vi "pih.hReadChannels-UandP-2018.vi"(0 "FPGA VI Reference In":refnum<k20>, 2 "SampleTime":sgl=0.0004, 3 "final channel selection":i64[][](array[numeric]), 4 "kbolott_and_volume":sgl[][](array[numeric]), 5 "Nsamples":u32, 7 "error in":errorcluster, 8 "Tau/dt":sgl[](array[numeric]), 9 "Scale(mV)":sgl[](array[numeric]), 11 "av power array":refnum<vi>, 15 "RawScal":sgl[](array[numeric]), 16 "SumScal":sgl[](array[numeric]), 17 "current P_rad sample":refnum<vi>) -> (1 "Fehler":bool, 20 "FPGA VI Reference Out":refnum<k20>, 21 "PowerArray":sgl[][](array[numeric]), 25 "RawArray":sgl[][](array[numeric]), 27 "error out":errorcluster)   [LabVIEW 2014]
doc: "startet das einlesen und führt dies bis n Samples aus\nHier mit FIFO und IRQ."
uses:
  <vilib>/Utility/error.llb/Error Cluster From Error Code.vi
  <vilib>/rvi/errors/niLvFpgaAdjustHostInterfaceError.vi
  <vilib>/RVI Host/nirviSupport.llb/nirviErrorClusterFromErrorCode.vi
  <vilib>/rvi/interface/nirviReadWriteControl/nirviReadWriteControl.xnode
  FPGA Bitfiles/W7XBolo2017_FPGATarget_fmain2014_9xlV3GyHFfo.lvbitx
  f_main_2014.vi
  <vilib>/rvi/interface/nirviMethod/nirviMethod.xnode
  NiFpgaLv.dll
  <vilib>/rvi/interface/nirviMethod/StockFPGA_InlinedMethodWaitForMultipleIRQ.vi
  <vilib>/FPGAPlugInAG/PCI-7813R/niLvFpga_WaitOnIrq_PCI-7813R.vi
  <vilib>/FPGAPlugInAG/PCI-7813R/niLvFpga_AcknowledgeIrq_PCI-7813R.vi
  <vilib>/FPGAPlugInAG/PCI-7813R/niLvFpga_ReadFifo_PCI-7813R.vi
  <vilib>/rvi/errors/niLvFpgaMergeErrorWithErrorCode.vi
panel:
  out "Array":sgl[](array[numeric])
  out "last sample":sgl[](array[numeric])
  out "x*2^n":dbl[](array[numeric])
  out "av array":dbl[](array[numeric])
  out "V_Cam":dbl format="%#_13g"
  out "new level of override":i32
  out "rt prad average array":dbl[][](array[numeric])
  out "rawarray":sgl[][](array[numeric])
  out "powerarray":sgl[][](array[numeric])
  out "current sample array":sgl[](array[numeric])
  in  "wait ms":i32
  out "column":i32
  out "channel index":i32
  out "sample":i32
  out "current P_rad [MW]":dbl
  out "elec. channel selected":i64
  out "sate":string
  out "element of channel\nand sample":sgl
  out "channel number":i64
  out "Elements Remaining":u32
  out "STOP?":bool
  out "Timed Out":bool
  # "Sampling"
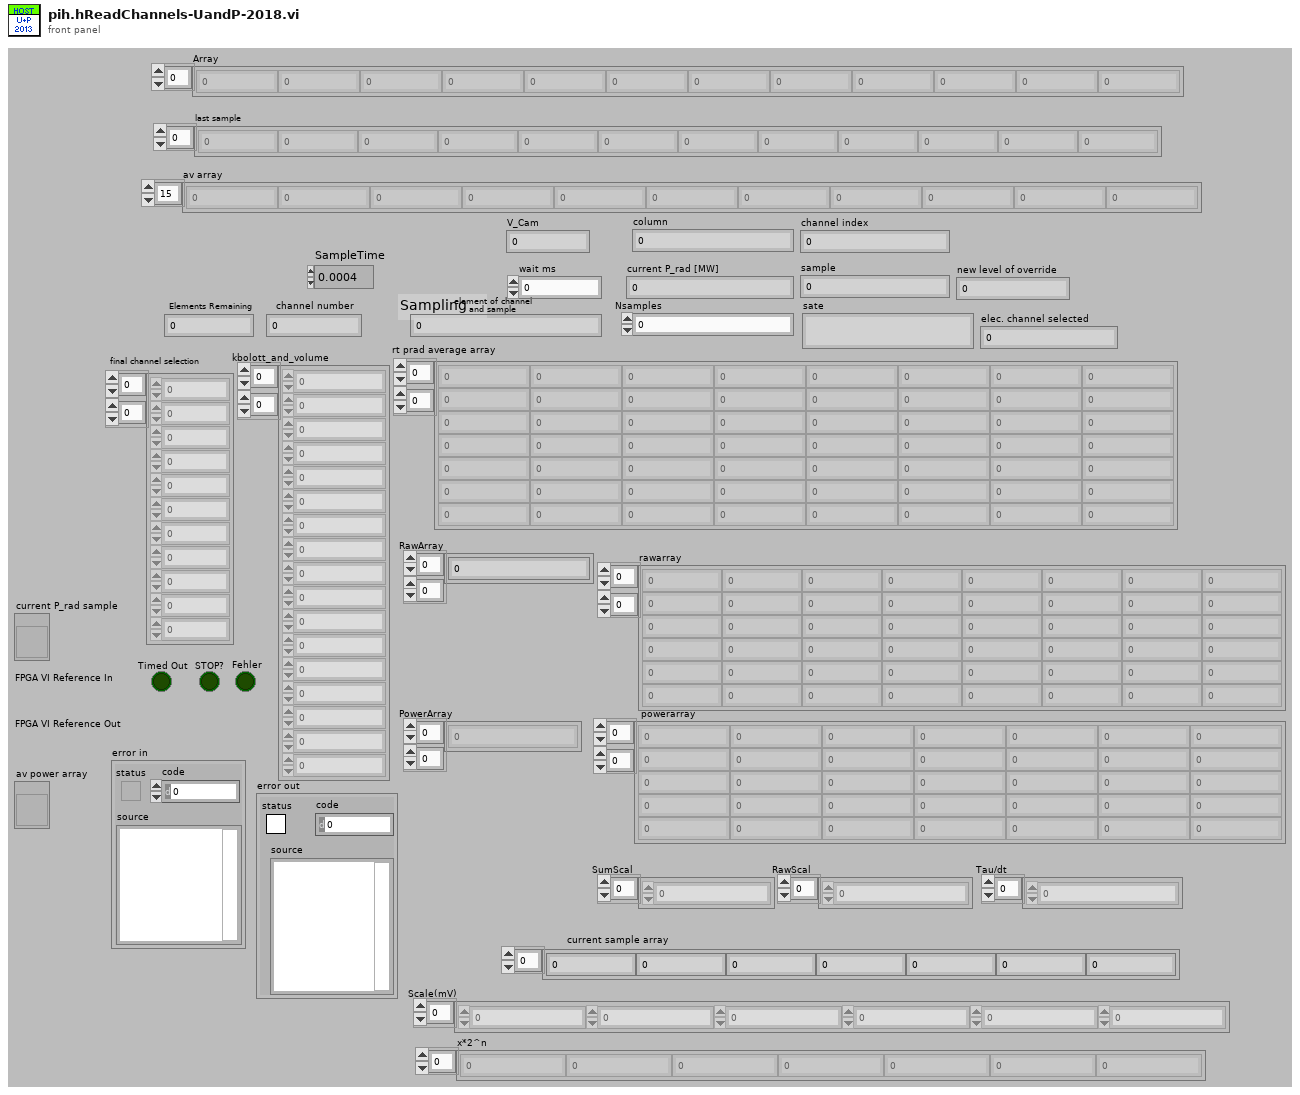
[diagram p1: front panel]
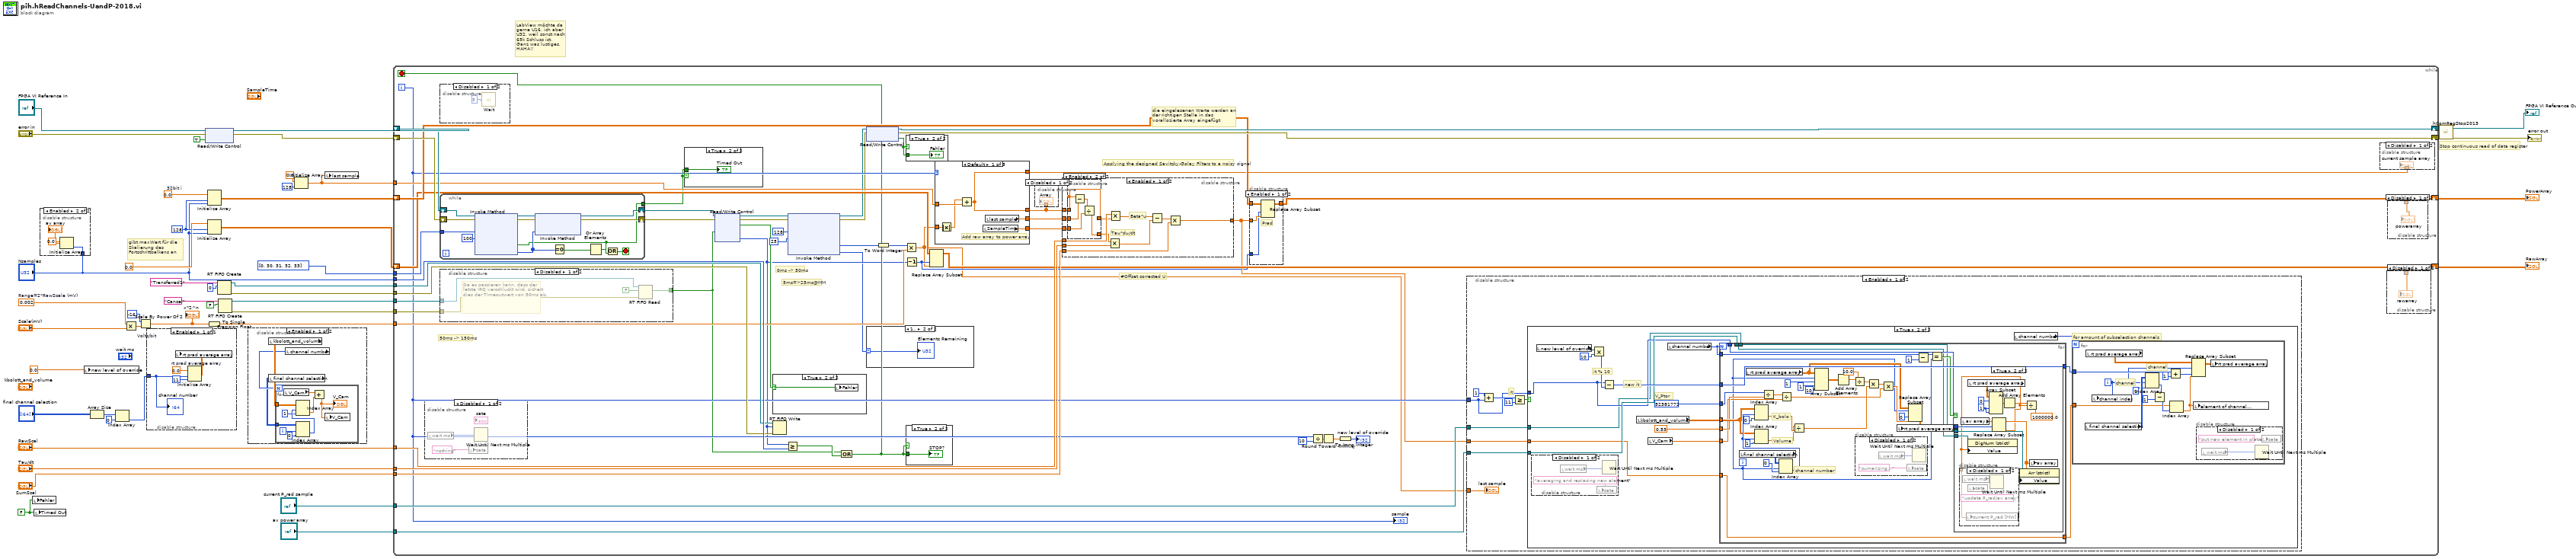
[diagram p0: block diagram]
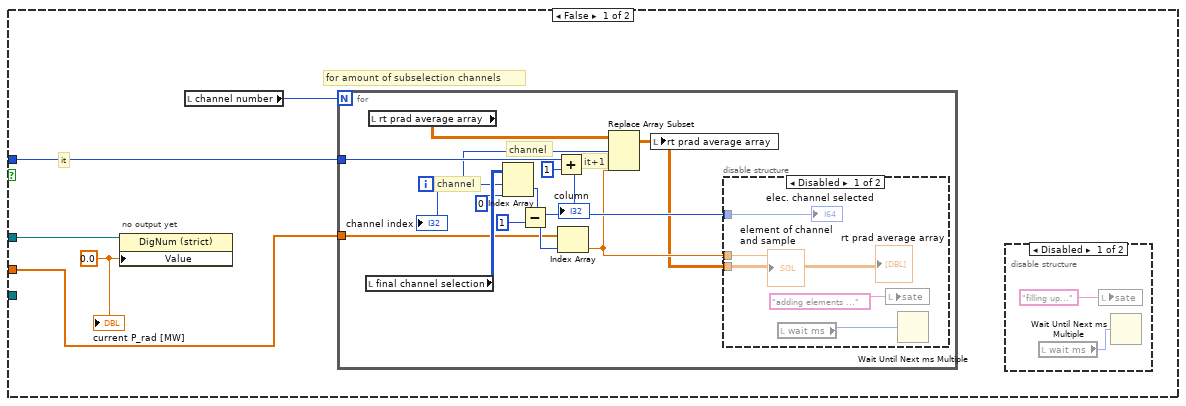
[diagram p5: hidden frame]
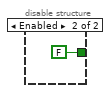
[diagram p17: hidden frame]
diagram:
  w19 = 0.002  # Range=2*RawScale (mV)
  w28 = 128 ("dimension size")
  w38 = sgl 0.0  # 32bit i
  w36 = FALSE
  # "Stop continuous read of data register"
  # "gibt maxWert für die Skalierung des Fortschrittbalkens an"
  # "LabView möchte da gerne U16, ich aber U32, weil sonst nach 65k Schluss ist. \nGanz was lustiges, HAHA!!"
  n1 = local write "Fehler"(w36) -> ()
  n2 = local write "Timed Out"(w36) -> ()
  n3 = disable-structure shown="Enabled" {
    disable-tunnel: "Nsamples" -> [_ w49]
    frame Disabled {
    }
    frame Enabled {
      n4 = Initialize Array(0.0 ("element"), w49) -> (→"av array":dbl[])
    }
  }
  n5 = local write "new level of override"(0.0 ("current level of override")) -> ()
  n6 = Array Size(array="final channel selection") -> (size(s)=w6:i32[])
  n7 = Index Array(array=w6, index=0) -> (element=w4:i32)
  n8 = Multiply(x=w19, y="Scale(mV)") -> (x*y=w20:dbl[])
  n9 = Scale By Power Of 2 "Volts/bit"(n=i16 -16, x=w20) -> (x*2^n=w21:dbl[])
  "x*2^n" <- w21
  n10 = disable-structure shown="Enabled" {
    disable-tunnel: w4 -> [w50]
    frame Enabled {
      n11 = Initialize Array "rt prad average array"(0.0 ("element"), w50, 11 ("dimension size")) -> (w51:dbl[][])
      n12 = local write "rt prad average array"(w51) -> ()
      "channel number" <- w50
    }
  }
  n13 = xnode "Read/Write Control"("FPGA VI Reference In"="FPGA VI Reference In", "error in"="error in", "ADCRead"=TRUE) -> ("FPGA VI Reference Out"=w25:refnum<k20>, "error out"=w24:errorcluster)
  n14 = Initialize Array(w38, w28, "Nsamples") -> (w37:sgl[][])
  n15 = Initialize Array(sgl 0.0, w28, "Nsamples") -> (w46:sgl[][])
  n16 = To Single Precision Float(number=w21) -> (single precision float=w18:sgl[])
  n17 = RT FIFO Create(0:"Transferred1" ("name (unnamed)"), 1:u32 0) -> (8:w43:refnum<k33>, 11:w42:errorcluster)  [unwired: 2 in, 5 out]
  n18 = RT FIFO Create(0:"Cancel" ("name (unnamed)"), 1:FALSE) -> (8:w40:refnum<k33>, 11:w39:errorcluster)  [unwired: 2 in, 5 out]
  n19 = disable-structure shown="Enabled" {
    frame Enabled {
      n20 = local read "kbolott_and_volume"() -> (w56:sgl[][])
      n21 = local read "final channel selection"() -> (w54:i64[][])
      n22 = local read "channel number"() -> (w55:i64)
      n23 = for {
        N: w55 -> [_]
        tunnel: w56 -> [w65]
        tunnel: w54 -> [w63]
        i -> [w64]
        n24 = local read "V_Cam"() -> (w61:dbl)
        n25 = Index Array(array=w63, index (row)=w64, index (col)=0 ("disabled index (col)")) -> (element=w59:i64)
        n26 = Index Array(array=w65, index (row)=w59, index (col)=1 ("disabled index (col)")) -> (element=w60:sgl)
        n27 = Add(x=w61, y=w60) -> (x+y=w57:dbl)
        "V_Cam" <- w57
        n28 = local write "V_Cam"(w57) -> ()
      }
    }
    frame Disabled {
    }
  }
  n29 = Initialize Array(sgl 0.0 ("element"), 128 ("dimension size")) -> (w1:sgl[])
  n30 = local write "last sample"(w1) -> ()
  n31 = while {
    tunnel: "Nsamples" -> [w112]
    shift-right: [w97] -> w29
    shift-left: w46 -> [w106]
    shift-right: [w113] -> w35
    shift-left: w25 -> [w116]
    shift-right: [w114] -> w34
    shift-left: w24 -> [w115]
    tunnel: w43 -> [w111]
    tunnel: w42 -> [w110]
    tunnel: w40 -> [w109]
    tunnel: w39 -> [w108]
    shift-right: [w98] -> w30
    shift-left: w37 -> [w107]
    tunnel: w18 -> [w105]
    tunnel: "Tau/dt" -> [w103]
    tunnel: "SumScal" -> [w104]
    tunnel: "RawScal" -> [w100]
    tunnel: i32[] [0, 30, 31, 32, 33] -> [w101]
    tunnel: "current P_rad sample" -> [w96]
    tunnel: "av power array" -> [w95]
    tunnel: w1 -> [w102]
    i -> [w94]
    stop <- w93 stop-if-true
    # "Applying the designed Savitzky-Golay Filters to a noisy signal"
    # "5ms=>25ms@MM"
    # "0ms -> 50ms"
    # "50ms -> 150ms"
    # "#Offset corrected U"
    # "die eingelesenen Werte werden an der richtigen Stelle in das vorallozierte Array eingefügt"
    n32 = disable-structure shown="Disabled" {
      frame Disabled {
        n33 = local read "wait ms"() -> (w238:i32)
        n34 = local write "sate"("nothing") -> ()
        n35 = Wait Until Next ms Multiple(millisecond multiple=w238) -> ()  [unwired: 1 out]
      }
      frame Enabled {
      }
    }
    n36 = disable-structure shown="Disabled" {
      frame Disabled {
        n37 = call "Wait"("Count(uSec)"=u32 5) -> ()  [unwired: 1 out]
      }
      frame Enabled {
      }
    }
    n38 = while {
      tunnel: [w243] -> w77
      shift-right: [w245] -> w73
      shift-left: w116 -> [w252]
      shift-right: [w244] -> w74
      shift-left: w115 -> [w251]
      tunnel: w101 -> [w249]
      stop <- w242 stop-if-true
      n39 = xnode "Invoke Method"("FPGA VI Reference In"=w252, "error in"=w251, "IRQ Number(s)"=w249, "Timeout (ms)"=100) -> ("FPGA VI Reference Out"=w246:refnum<k20>, "error out"=w247:errorcluster, "Timed Out"=w243:bool, "IRQ(s) Asserted"=w248:i32[])
      n40 = xnode "Invoke Method"("FPGA VI Reference In"=w246, "error in"=w247, "IRQ Number(s)"=w248) -> ("FPGA VI Reference Out"=w245:refnum<k20>, "error out"=w244:errorcluster)
      n41 = Equal To 0?(x=w248) -> (x = 0?=w241:bool[])
      n42 = Or Array Elements(Boolean array=w241) -> (logical OR=w240:bool)
      n43 = Or(x=w240, y=w243) -> (x .or. y?=w242:bool)
    }
    n44 = disable-structure shown="Disabled" {
      disable-tunnel: [w258 FALSE] -> w90
      disable-tunnel: w109 -> [w257 _]
      disable-tunnel: w108 -> [w256 _]
      frame Disabled {
        # "Da es passieren kann, dass der letzte IRQ verschluckt wird, sichert dies der Timeoutwert von 50ms ab."
        n45 = RT FIFO Read(0:w257, 1:FALSE ("element"), 3:w256) -> (9:w258:bool)  [unwired: 5 out]
      }
      frame Enabled {
      }
    }
    n46 = case shown="True" w77 {
      tunnel: w77 -> [_ w266]
      frame False {
      }
      frame True {
        "Timed Out" <- w266
      }
    }
    n47 = xnode "Read/Write Control"("FPGA VI Reference In"=w73, "error in"=w74, "cancel"=w90) -> ("FPGA VI Reference Out"=w88:refnum<k20>, "error out"=w87:errorcluster, "Timeout"=w89:bool, "ScanID"=w85:u32)
    n48 = case shown="True" w89 {
      selector: w89 -> [_ w303]
      frame False {
      }
      frame True {
        n49 = local write "Fehler"(w303) -> ()
      }
    }
    n50 = RT FIFO Write(0:w111, 1:w85, 3:w110) -> ()  [unwired: 1 in, 5 out]
    n51 = Greater Or Equal?(x=w85, y=w112) -> (x >= y?=w91:bool)
    n52 = xnode ("Invoke Method")("FPGA VI Reference In"=w88, "error in"=w87, "Number of Elements"=u32 128, "Timeout (ms)"=25 ("Timeout")) -> ("FPGA VI Reference Out"=w80:refnum<k20>, "error out"=w79:errorcluster, "Data"=w82:u32[], "Elements Remaining"=w76:u32)
    n53 = Compound Arithmetic op=OR(w90, w91) -> (w93:bool)
    n54 = xnode "Read/Write Control"("FPGA VI Reference In"=w80, "error in"=w79) -> ("FPGA VI Reference Out"=w113:refnum<k20>, "error out"=w114:errorcluster, "Fifo-Fehler"=w75:bool)
    n55 = case shown="1.." w76 {
      selector: w76 -> [_ w265]
      frame 0, Default {
      }
      frame 1.. {
        "Elements Remaining" <- w265
      }
    }
    n56 = To Word Integer(number=w82) -> (16bit integer=w81:i16[])
    n57 = Multiply(x=w81, y=w105) -> (x*y=w66:sgl[])
    n58 = Decrement(x=w85) -> (x-1=w86:u32)
    n59 = case shown="True" w75 {
      tunnel: w75 -> [_ w254]
      frame False {
      }
      frame True {
        "Fehler" <- w254
      }
    }
    n60 = case shown="True" w93 {
      tunnel: w93 -> [_ w253]
      frame False {
      }
      frame True {
        "STOP?" <- w253
      }
    }
    n61 = Replace Array Subset(array=w106, new element=w66, index (col)=w86) -> (w97:sgl[][])  [unwired: 1 in]
    n62 = case shown="Default" w94 {
      tunnel: w66 -> [w294 _ w301]
      tunnel: [w295 w299 w302] -> w99
      tunnel: w102 -> [w296 w297 w302]
      tunnel: [w295 w297 w300] -> w78
      tunnel: [w292 _ _] -> w68
      tunnel: [w291 _ _] -> w67
      frame Default {
        # "Add raw array to power array"
        n63 = Absolute Value(x=w294) -> (abs(x)=w293:sgl[])
        n64 = Add(x=w293, y=w296) -> (x+y=w295:sgl[])
        n65 = local read "SampleTime"() -> (w291:sgl)
        n66 = local read "last sample"() -> (w292:sgl[])
      }
      frame -1 {
        n67 = Divide(x=w297, y=sgl 60.0) -> (x/y=w299:sgl[])
      }
      frame -2 {
        n68 = Subtract(x=w301, y=w302) -> (x-y=w300:sgl[])
      }
    }
    n69 = disable-structure shown="Disabled" {
      disable-tunnel: w78 -> [w117 _]
      frame Disabled {
        "Array" <- w117
      }
      frame Enabled {
      }
    }
    n70 = disable-structure shown="Enabled" {
      disable-tunnel: w104 -> [w278 _]
      disable-tunnel: w100 -> [w277 _]
      disable-tunnel: w103 -> [w276 _]
      disable-tunnel: [w275 w289] -> w92
      disable-tunnel: w78 -> [w274 w289]
      disable-tunnel: w68 -> [w268 _]
      disable-tunnel: w67 -> [w267 _]
      frame Enabled {
        # "Beta*u"
        # "Tau*du/dt"
        n71 = disable-structure shown="Enabled" {
          disable-tunnel: w274 -> [w283 w288]
          disable-tunnel: [w282 w284] -> w271
          disable-tunnel: [w279 w288] -> w269
          disable-tunnel: w268 -> [_ w287]
          disable-tunnel: w267 -> [_ w285]
          frame Disabled {
            n72 = call "Savitzky Golay Filter PtByPt with Derivative861.vi"("order polynomial"=2, "side points"=31, "x"=w283) -> ("Filtered Derivative"=w282:dbl[], "Filtered x"=w279:dbl[])  [unwired: 1 in, 6 out]
          }
          frame Enabled {
            n73 = Subtract(x=w288, y=w287) -> (x-y=w286:sgl[])
            n74 = Divide(x=w286, y=w285) -> (x/y=w284:sgl[])
          }
        }
        n75 = Multiply(x=w271, y=w276) -> (x*y=w270:sgl[])
        n76 = Multiply(x=w277, y=w269) -> (x*y=w273:sgl[])
        n77 = Subtract(x=w273, y=w270) -> (x-y=w272:sgl[])
        n78 = Multiply(x=w272, y=w278) -> (x*y=w275:sgl[])
      }
      frame Disabled {
      }
    }
    n79 = disable-structure shown="Enabled" {
      disable-tunnel: w107 -> [w263 w264]
      disable-tunnel: [w262 w264] -> w98
      disable-tunnel: w86 -> [w260 _]
      disable-tunnel: w92 -> [w261 _]
      frame Enabled {
        # "Prad"
        n80 = Replace Array Subset(array=w263, new element=w261, index (col)=w260) -> (w262:sgl[][])  [unwired: 1 in]
      }
      frame Disabled {
      }
    }
    n81 = Divide(x=w94, y=10) -> (x/y=w71:dbl)
    n82 = Round Toward -Infinity(1:w71) -> (0:w70:dbl)
    n83 = To Long Integer(number=w70) -> (32bit integer=→"new level of override":i32)
    n84 = disable-structure shown="Enabled" {
      disable-tunnel: w94 -> [w119 _]
      disable-tunnel: w96 -> [w122 _]
      disable-tunnel: w95 -> [w121 _]
      disable-tunnel: w92 -> [w120 _]
      disable-tunnel: w66 -> [w118 _]
      frame Enabled {
        # "it"
        n85 = Add(x=1, y=w119) -> (x+y=w123:i32)
        n86 = Greater Or Equal?(x=w123, y=11) -> (x >= y?=w125:bool)
        n87 = case shown="True" w125 {
          tunnel: w119 -> [w127 w154]
          tunnel: w122 -> [w130 w153]
          tunnel: w121 -> [_ w155]
          tunnel: w120 -> [w128 w152]
          frame False {
            w129 = 0.0 ("Value")
            # "it"
            # "for amount of subselection channels"
            # "no output yet"
            n88 = property class="DigNum (strict)"(reference=w130, "Value"=w129) -> ()  [unwired: 1 in, 2 out]
            n89 = local read "channel number"() -> (w131:i64)
            n90 = for {
              N: w131 -> [_]
              tunnel: w127 -> [w140]
              tunnel: w128 -> [w137]
              i -> [w134]
              # "channel"
              # "channel"
              # "it+1"
              n91 = local read "final channel selection"() -> (w146:i64[][])
              n92 = local read "rt prad average array"() -> (w138:dbl[][])
              n93 = Index Array(array=w146, index (row)=w134, index (col)=0 ("disabled index (col)")) -> (element=w142:i64)
              n94 = Subtract(x=w142, y=i64 1) -> (x-y=w139:i64)
              n95 = Add(x=w140, y=1) -> (x+y=w143:i32)
              "column" <- w143
              n96 = Index Array(array=w137, index=w139) -> (element=w136:sgl)
              n97 = Replace Array Subset(array=w138, new element=w136, index (row)=w134, index (col)=w143) -> (w135:dbl[][])
              n98 = local write "rt prad average array"(w135) -> ()
              n99 = disable-structure shown="Disabled" {
                disable-tunnel: w139 -> [w150 _]
                disable-tunnel: w136 -> [w148 _]
                disable-tunnel: w135 -> [w147 _]
                frame Disabled {
                  n100 = local read "wait ms"() -> (w149:i32)
                  n101 = local write "sate"("adding elements ...") -> ()
                  n102 = Wait Until Next ms Multiple(millisecond multiple=w149) -> ()  [unwired: 1 out]
                  "element of channel\nand sample" <- w148
                  "elec. channel selected" <- w150
                  "rt prad average array" <- w147
                }
                frame Enabled {
                }
              }
              "channel index" <- w134
            }
            n103 = disable-structure shown="Disabled" {
              frame Disabled {
                n104 = local read "wait ms"() -> (w132:i32)
                n105 = local write "sate"("filling up...") -> ()
                n106 = Wait Until Next ms Multiple(millisecond multiple=w132) -> ()  [unwired: 1 out]
              }
              frame Enabled {
              }
            }
            "current P_rad [MW]" <- w129
          }
          frame True {
            # "V_Ptor"
            # "new it"
            # "it % 10"
            # "for amount of subselection channels"
            n107 = disable-structure shown="Disabled" {
              frame Disabled {
                n108 = local read "wait ms"() -> (w168:i32)
                n109 = local write "sate"("averaging and replacing new element") -> ()
                n110 = Wait Until Next ms Multiple(millisecond multiple=w168) -> ()  [unwired: 1 out]
              }
              frame Enabled {
              }
            }
            n111 = local read "new level of override"() -> (w166:i32)
            n112 = Multiply(x=w166, y=10) -> (x*y=w164:i32)
            n113 = Subtract(x=w154, y=w164) -> (x-y=w162:i32)
            n114 = local read "kbolott_and_volume"() -> (w163:sgl[][])
            n115 = local read "V_Cam"() -> (w159:dbl)
            n116 = local read "channel number"() -> (w157:i64)
            n117 = for {
              N: w157 -> [_]
              tunnel: w163 -> [w199]
              tunnel: [w205] -> w158
              tunnel: w152 -> [w205]
              tunnel: [w204] -> w156
              tunnel: w162 -> [w204]
              tunnel: 52381772 -> [w195]
              tunnel: 0.53 -> [w194]
              tunnel: w159 -> [w192]
              tunnel: w157 -> [w172]
              tunnel: w154 -> [w175]
              tunnel: w155 -> [w174]
              tunnel: w153 -> [w170]
              i -> [w177]
              # "K_bolo"
              # "Volume"
              # "channel number"
              n118 = local read "final channel selection"() -> (w203:i64[][])
              n119 = local read "rt prad average array"() -> (w181:dbl[][])
              n120 = Divide(x=w195, y=w194) -> (x/y=w193:dbl)
              n121 = Index Array(array=w203, index (row)=w177, index (col)=0 ("disabled index (col)")) -> (element=w200:i64)
              n122 = Index Array(array=w199, index (row)=w200, index (col)=0 ("disabled index (col)")) -> (element=w197:sgl)
              n123 = Index Array(array=w199, index (row)=w200, index (col)=1 ("disabled index (col)")) -> (element=w196:sgl)
              n124 = Divide(x=w193, y=w192) -> (x/y=w182:dbl)
              n125 = Divide(x=w196, y=w197) -> (x/y=w184:sgl)
              n126 = Array Subset(array=w181, index (row)=w177, length (row)=1, index (col)=1 ("index"), length (col)=10 ("length")) -> (w188:dbl[][])
              n127 = Add Array Elements(numeric array=w188) -> (sum=w187:dbl)
              n128 = Divide(x=w187, y=10.0) -> (x/y=w185:dbl)
              n129 = disable-structure shown="Disabled" {
                frame Disabled {
                  n130 = local read "wait ms"() -> (w207:i32)
                  n131 = local write "sate"("sumarizing...") -> ()
                  n132 = Wait Until Next ms Multiple(millisecond multiple=w207) -> ()  [unwired: 1 out]
                }
                frame Enabled {
                }
              }
              n133 = Multiply(x=w185, y=w184) -> (x*y=w183:dbl)
              n134 = Multiply(x=w183, y=w182) -> (x*y=w180:dbl)
              n135 = Replace Array Subset(array=w181, new element=w180, index (row)=w177, index (col)=0 ("disabled index (col)")) -> (w178:dbl[][])
              n136 = local write "rt prad average array"(w178) -> ()
              n137 = Subtract(x=w172, y=i64 1) -> (x-y=w173:i64)
              n138 = Equal?(x=w173, y=w177) -> (x = y?=w176:bool)
              n139 = case shown="True" w176 {
                tunnel: w175 -> [_ w214]
                tunnel: w174 -> [_ w213]
                tunnel: w170 -> [_ w212]
                frame False {
                }
                frame True {
                  w218 = 1 ("index")
                  n140 = local read "av array"() -> (w215:dbl[])
                  n141 = local read "rt prad average array"() -> (w216:dbl[][])
                  n142 = Array Subset(array=w216, index (row)=0 ("index"), index (col)=w218, length (col)=w218) -> (w219:dbl[][])  [unwired: 1 in]
                  n143 = Add Array Elements(numeric array=w219) -> (sum=w210:dbl)
                  n144 = Divide(x=w210, y=1000000.0) -> (x/y=w208:dbl)
                  n145 = disable-structure shown="Disabled" {
                    disable-tunnel: w208 -> [w220 _]
                    frame Disabled {
                      n146 = local read "wait ms"() -> (w222:i32)
                      n147 = local write "current P_rad [MW]"(w220) -> ()
                      n148 = local write "sate"("update P_rad/av array") -> ()
                      n149 = Wait Until Next ms Multiple(millisecond multiple=w222) -> ()  [unwired: 1 out]
                    }
                    frame Enabled {
                    }
                  }
                  n150 = property class="DigNum (strict)"(reference=w212, "Value"=w208) -> ()  [unwired: 1 in, 2 out]
                  n151 = Replace Array Subset(array=w215, new element=w208, index=w214) -> (w211:dbl[])
                  n152 = property class="Arr (strict)"(reference=w213, "Value"=w211) -> ()  [unwired: 1 in, 2 out]
                  n153 = local write "av array"(w211) -> ()
                }
              }
            }
            n154 = local read "channel number"() -> (w167:i64)
            n155 = for {
              N: w167 -> [_]
              tunnel: w156 -> [w229]
              tunnel: w158 -> [w226]
              i -> [w223]
              # "channel"
              # "channel"
              n156 = local read "final channel selection"() -> (w235:i64[][])
              n157 = local read "rt prad average array"() -> (w227:dbl[][])
              n158 = local write "channel index"(w223) -> ()
              n159 = Index Array(array=w235, index (row)=w223, index (col)=0 ("disabled index (col)")) -> (element=w231:i64)
              n160 = Subtract(x=w231, y=i64 1) -> (x-y=w228:i64)
              n161 = Add(x=w229, y=1) -> (x+y=w232:i32)
              n162 = Index Array(array=w226, index=w228) -> (element=w224:sgl)
              n163 = Replace Array Subset(array=w227, new element=w224, index (row)=w223, index (col)=w232) -> (w225:dbl[][])
              n164 = local write "element of channel\nand sample"(w224) -> ()
              n165 = disable-structure shown="Disabled" {
                frame Disabled {
                  n166 = local read "wait ms"() -> (w236:i32)
                  n167 = Wait Until Next ms Multiple(millisecond multiple=w236) -> ()  [unwired: 1 out]
                  n168 = local write "sate"("put new element in place") -> ()
                }
                frame Enabled {
                }
              }
              n169 = local write "rt prad average array"(w225) -> ()
            }
          }
        }
        "last sample" <- w118
      }
      frame Disabled {
      }
    }
    n170 = disable-structure shown="Disabled" {
      disable-tunnel: w99 -> [w306 _]
      frame Disabled {
        "current sample array" <- w306
      }
      frame Enabled {
      }
    }
    n171 = disable-structure shown="Disabled" {
      disable-tunnel: w97 -> [w304 _]
      frame Disabled {
        "rawarray" <- w304
      }
      frame Enabled {
      }
    }
    n172 = disable-structure shown="Disabled" {
      disable-tunnel: w98 -> [w305 _]
      frame Disabled {
        "powerarray" <- w305
      }
      frame Enabled {
      }
    }
    "sample" <- w94
  }
  "RawArray" <- w29
  "PowerArray" <- w30
  n173 = call "hComRegStop2013.vi"("error in"=w34, "FPGA VI Reference In"=w35) -> ("error out"=→"error out":errorcluster, "FPGA VI Reference Out"=→"FPGA VI Reference Out":refnum<k20>)  [unwired: 3 in, 1 out]
